vi "ModeConfig.vi"(8 "error in (no error)":errorcluster, 10 "Drive State":T1, 11 "Tank Drive in":refnum<class "Tank Drive.lvclass">) -> (0 "error out":errorcluster, 3 "Tank Drive out":refnum<class "Tank Drive.lvclass">)   [LabVIEW 2019, in "Drive.lvlib" / "Tank Drive.lvclass"]
uses:
  Tank Drive.lvclass
  Controls/Drive State.ctl
  Tank Drive.lvclass/Tank Drive.ctl
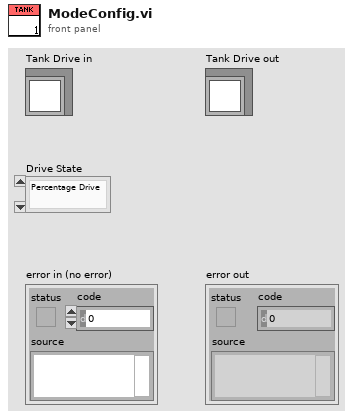
[diagram p1: front panel]
types:
  T1 = typedef "Drive.lvlib/Tank Drive.lvclass/Drive State.ctl" = enum16{"Percentage Drive", "Velocity Drive", "PID to Position", "Motion Profile"}
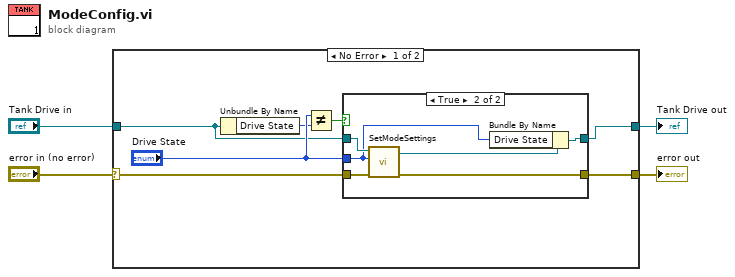
[diagram p0: block diagram]
diagram:
  n1 = case shown="No Error" "error in (no error)" {
    selector: "error in (no error)" -> [w11 w21]
    tunnel: [w10 w21] -> w3
    tunnel: "Tank Drive in" -> [w8 w20]
    tunnel: [w7 w20] -> w1
    frame No Error {
      n2 = Unbundle By Name(w8) -> ("Drive State"=w6:T1)
      n3 = Not Equal?(x="Drive State", y=w6) -> (x != y?=w5:bool)
      n4 = case shown="True" w5 {
        tunnel: w11 -> [w13 w19]
        tunnel: [w13 w18] -> w10
        tunnel: "Drive State" -> [_ w14]
        tunnel: [w12 w15] -> w7
        tunnel: w8 -> [w12 w17]
        frame False {
        }
        frame True {
          n5 = call "SetModeSettings.vi"("error in (no error)"=w19, "Drive State"=w14, "Tank Drive in"=w17) -> ("error out"=w18:errorcluster, "Tank Drive out"=w16:refnum<class "Tank Drive.lvclass">)  [unwired: 7 in]
          n6 = Bundle By Name(cluster=w16, "Drive State"=w14) -> (w15:refnum<class "Tank Drive.lvclass">)
        }
      }
    }
    frame Error {
    }
  }
  "error out" <- w3
  "Tank Drive out" <- w1
